vi "Signal acquisition on external trigger.vi"() -> ()   [LabVIEW 2010]
doc: "This example shows how to acquire 16k samples of signal on fast analog inputs. Signal will be acquired when the external trigger condition is meet. Time length of the acquired signal depends on the time scale of a buffer that can be set with a decimation factor. Decimations and time scales of a buffer are given in the table below. Voltage range of fast analog inputs on the Red Pitaya depends on gain setting that can be set by jumpers. HV setting is for input range to ±20V, while LV sets input range to ±1V."
uses:
  RedPitaya.lvlib
panel:
  in  "Trigger Level (0 V)":dbl=1.1 min=-20.0 max=20.1
  in  "Delay (# Samples)":i32 max=16348
  in  "Decimation":u32(ring)=8 items=["65536"=65536, "8192"=8192, "1024"=1024, "64"=64, "8"=8, "1"=1]
  in  "IP address":string="192.168.1.100"
  out "Waveform Graph":dbl[](graph)
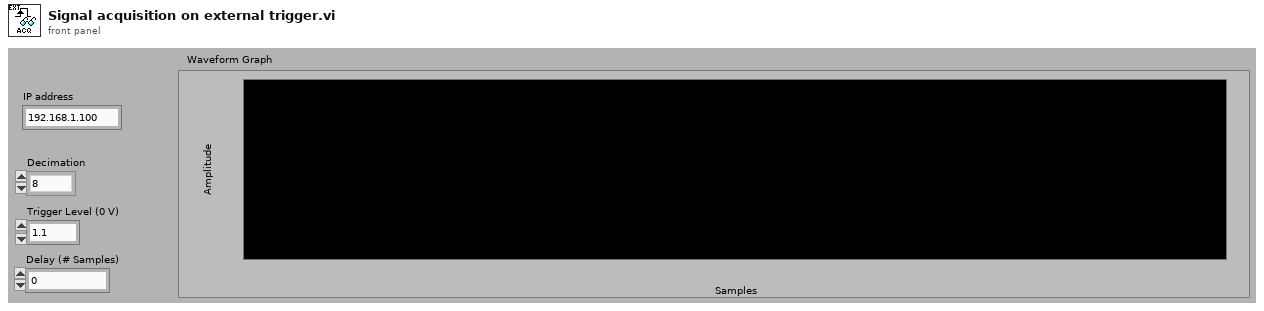
[diagram p1: front panel]
types:
  T1 = enum16{"Disabled", "Now", "Ch1 positive edge", "Ch1 negative edge", "Ch2 positive edge", "Ch2 negative edge", "external positive ege", "external negative edge", "AWG positive edge", "AWG negative edge"}
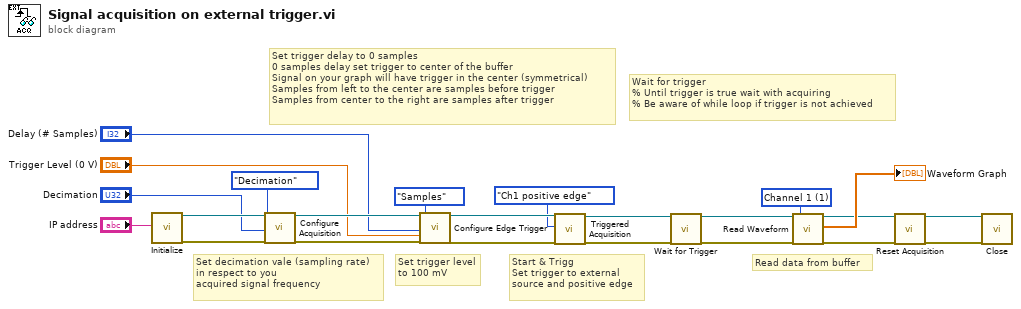
[diagram p0: block diagram]
diagram:
  w23 = u16 1 items=["Channel 1"=1, "Channel 2"=2] ("Channel (1|2)")
  # "Read data from buffer"
  # "Start & Trigg\nSet trigger to external\nsource and positive edge"
  # "Wait for trigger\n% Until trigger is true wait with acquiring\n% Be aware of while loop if trigger is not achieved"
  # "Set trigger delay to 0 samples\n0 samples delay set trigger to center of the buffer\nSignal on your graph will have trigger in the center (symmetrical)\nSamples from left to the center are samples before trigger \nSamples from center to the right are samples after trigger"
  # "Set trigger level\nto 100 mV"
  # "Set decimation vale (sampling rate)\nin respect to you \nacquired signal frequency"
  n1 = call "Initialize.vi"("IP address"="IP address") -> ("RedPitaya connection out"=w9:refnum<k5>, "error out"=w8:errorcluster)  [unwired: 17 in]
  n2 = call "Configure Acquisition.vi"("RedPitaya connection in"=w9, "Decimation/Sampling Rate"=enum16{"", "Sampling rate", "Decimation"}."Decimation", "Decimation"="Decimation", "error in"=w8) -> ("RedPitaya connection out"=w10:refnum<k5>, "error out"=w7:errorcluster)  [unwired: 14 in]
  n3 = call "Configure Edge Trigger.vi"("RedPitaya connection in"=w10, "Trigger Delay mode"=enum16{"", "Samples", "Nanoseconds"}."Samples", "Delay (# Samples)"="Delay (# Samples)", "Trigger Level (0 V)"="Trigger Level (0 V)", "error in"=w7) -> ("RedPitaya connection out"=w21:refnum<k5>, "error out"=w20:errorcluster)  [unwired: 13 in]
  n4 = call "Triggered Acquisition.vi"("RedPitaya TCP connection in"=w21, "Trigger Mode"=T1."Ch1 positive edge", "error in"=w20) -> ("RedPitaya TCP connection out"=w18:refnum<k5>, "error out"=w15:errorcluster)  [unwired: 15 in]
  n5 = call "Wait for Trigger.vi"("RedPitaya TCP connection in"=w18, "error in"=w15) -> ("RedPitaya TCP connection out"=w17:refnum<k5>, "error out"=w16:errorcluster)  [unwired: 16 in]
  n6 = call "Read Waveform.vi"("RedPitaya TCP Connection in"=w17, "error in"=w16, "Channel #"=w23) -> ("RedPitaya TCP Connection out"=w14:refnum<k5>, "Measurement Array"=→"Waveform Graph":dbl[], "error out"=w12:errorcluster)  [unwired: 14 in]
  n7 = call "Reset Acquisition.vi"("RedPitaya connection in"=w14, "error in"=w12) -> ("RedPitaya connection out"=w13:refnum<k5>, "error out"=w11:errorcluster)  [unwired: 16 in]
  n8 = call "Close.vi"("RedPitaya connection in"=w13, "error in"=w11) -> ()  [unwired: 17 in, 1 out]
